vi "InterceptBall.vi"(6 "passer tactic":T1=enum."PenaltyAttacker", 7 "firstCall":bool, 8 "error in (no error)":errorcluster, 9 "Robot":refnum<class "Robot.lvclass">, 10 "Game":refnum<class "Game.lvclass">, 11 "ShootTactic in":refnum<class "ShootTactic.lvclass">) -> (0 "error out":errorcluster, 2 "robot out":refnum<class "Robot.lvclass">, 3 "ShootTactic out":refnum<class "ShootTactic.lvclass">)   [LabVIEW 2023]
uses:
  Utilities_class/Utilities.lvclass
  WaitBallTrajSkill_class/WaitBallTrajSkill.lvclass
  Robot_class/robotKickToStates.ctl
  Robot_class/tactics.ctl
  Robot_class/roles.ctl
  Robot_class/Robot.lvclass
  Ally_class/Ally.lvclass
  Parameters_class/Parameters.lvclass
  Game_class/Game.lvclass
  Zone_class/Zone.lvclass
  Ball_class/Ball.lvclass
  Field_class/Field.lvclass
  C:/Users/ebert/Desktop/roboime/SSL_AI/Skill_class/Skill.lvclass
  C:/Users/ebert/Desktop/roboime/SSL_AI/WaitBallTrajSkill_class/WaitBallTrajSkill.lvclass
  ShootTactic.lvclass
  C:/Users/ebert/Desktop/roboime/SSL_AI/Tactic_class/Tactic.lvclass
  C:/Users/ebert/Desktop/roboime/SSL_AI/ShootTactic_class/ShootTactic.lvclass
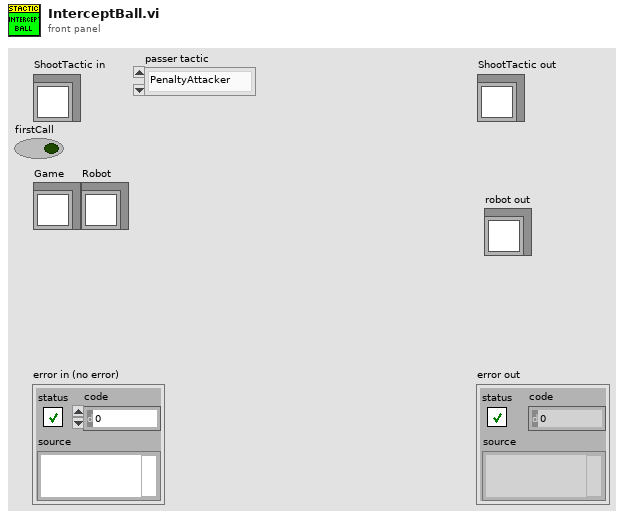
[diagram p1: front panel]
types:
  T1 = typedef "tactics.ctl" = enum16{"GoToBallPlacementPosition", "PlaceBall", "GoToBallPlacement", "5Robots", "BallPlacementEnemy", "ReceivePassInFuturePoint", "Roller", "PrepareRollToPassRollerGoTo", "PrepareRollToPassReceiverGoTo", "WaitRoll", "PositionToRoll", "PenaltyAttacker", "PassObserver", "PenaltyDefense", "TableReceiverTactic", "Test", "DefendGoal", "Marker", "FollowAttacker", "DefendArea", "Shoot", "AttackerAimGoal", "AttackerBallOutOfField", "AttackerBlock", "AttackerStop", "Duelist", "Halt", "ZigZag", "GoTo", "Timeout", "KickToBestRobot", "KickToPassReceiver", "PositionToReceivePass", "WaitPass", "GoToTarget"}
  T2 = typedef "roles.ctl" = enum16{"SimpleBallPlacement", "BallPlacementAllyPasser", "BallPlacementAllyReceiver", "BallPlacementEnemy", "5Robots5th", "PassBestReceiver", "5Robots4th", "5Robots3rd", "5Robots2nd", "5Robots1st", "PassBestRobot", "WaitPass", "ABCThirdKicker", "ABCFirstKicker", "ABCSecondKicker", "Tabler", "TableFinalizer", "PrepareRollToPassRoller", "PrepareRollToPassReceiver", "SimplePassRoll", "SimplePassRollReceiver", "PenaltyDefense", "PreparePassReceiver 2", "PreparePassReceiver 1", "PassObserver", "Timeout", "Goto", "ZigZag", "None", "BallOutOfField", "DefenderArea", "Duelist", "AttackerStop", "FollowAttacker", "KeeperRole", "KickPenalty", "AttackerAimGoal", "AttackerBlock", "Marker", "Halt", "Shoot", "PassKicker", "PassReceiver", "TestRole", "PenaltyAttacker"}
  T3 = typedef "robotKickToStates.ctl" = enum16{"shootFromDirect", "avoidCollideBall", "goToBackBall", "none", "walk", "turn", "turnAntiClockWise", "turnClockwise", "oldKickToShoot", "oldKickToGoToBackBall", "shoot"}
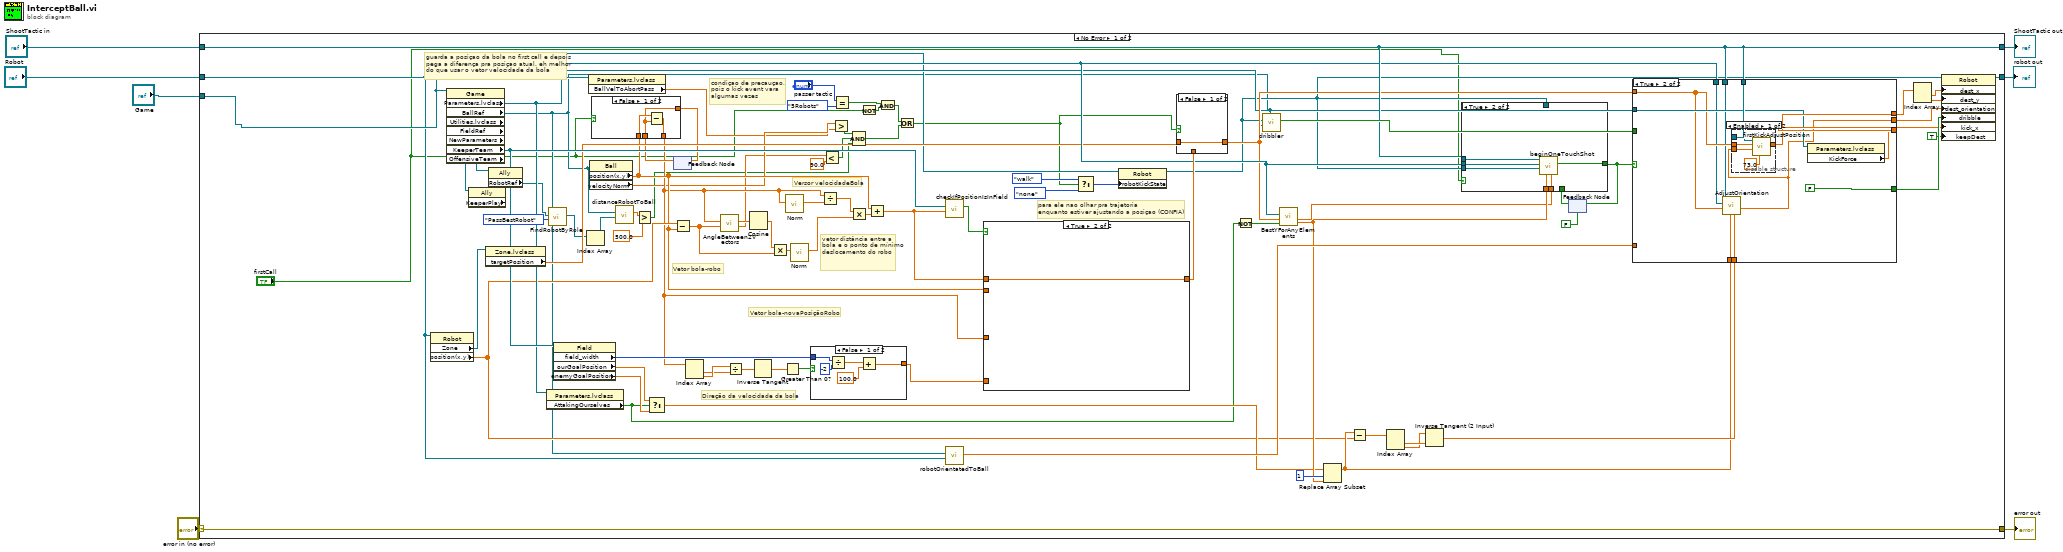
[diagram p0: block diagram]
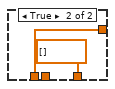
[diagram p2: hidden frame]
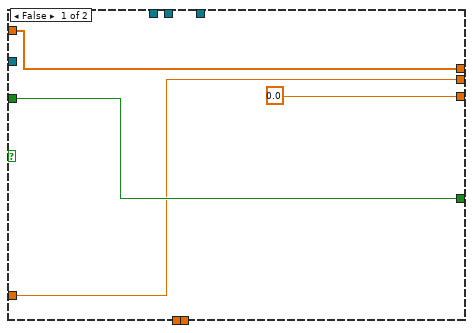
[diagram p4: hidden frame]
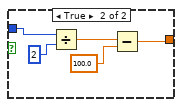
[diagram p7: hidden frame]
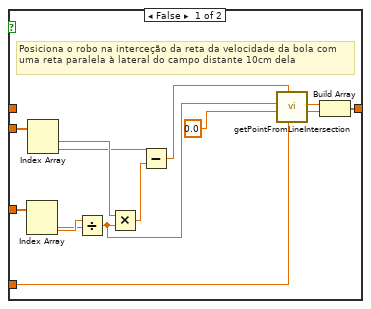
[diagram p8: hidden frame]
diagram:
  n1 = case shown="No Error" "error in (no error)" {
    selector: "error in (no error)" -> [w93 w155]
    tunnel: [w93 w155] -> w6
    tunnel: [w56 w154] -> w4
    tunnel: "ShootTactic in" -> [w56 w154]
    tunnel: "Robot" -> [w40 _]
    tunnel: "Game" -> [w55 _]
    tunnel: [w92 _] -> w2
    frame No Error {
      # "guarda a posiçao da bola no first call e depois\npega a diferença pra posiçao atual. eh melhor\ndo que usar o vetor velocidade da bola"
      # "condiçao de precauçao,\npois o kick event vara \nalgumas vezes"
      # "para ele nao olhar pra trajetoria \nenquanto estiver ajustando a posiçao (CONFIA)"
      # "vetor distância entre a bola e o ponto de mínimo deslocamento do robo"
      # "Versor velocidadeBola"
      # "Direção da velocidade da bola"
      # "Vetor bola-novaPosiçãoRobo"
      # "Vetor bola-robo"
      n2 = property class="Robot"(reference=w40) -> ("Zone"=w43:refnum<class "Zone.lvclass">, "position(x,y)"=w44:dbl[])  [unwired: 1 in, 2 out]
      n3 = property class="Game" props=["Parameters.lvclass", "BallRef", "Utilities.lvclass", "FieldRef", "NewParameters", "KeeperTeam", "OffensiveTeam"](reference=w55) -> ("Parameters.lvclass"=w45:refnum<class "Parameters.lvclass">, "BallRef"=w12:refnum<class "Ball.lvclass">, "FieldRef"=w78:refnum<class "Field.lvclass">, "KeeperTeam"=w68:refnum<class "Ally.lvclass">, "OffensiveTeam"=w16:refnum<class "Ally.lvclass">)  [unwired: 1 in, 4 out]
      n4 = property class="Ally" props=["KeeperPlay"](reference=w68) -> ()  [unwired: 1 in, 3 out]
      n5 = property class="Zone.lvclass"(reference=w43) -> ("targetPosition"=w42:dbl[])  [unwired: 1 in, 2 out]
      n6 = property class="Ally"(reference=w16) -> ("RobotRef"=w15:refnum<class "Robot.lvclass">[])  [unwired: 1 in, 2 out]
      n7 = property class="Parameters.lvclass"(reference=w45) -> ("AttakingOurselves"=w49:bool)  [unwired: 1 in, 2 out]
      n8 = call "FindRobotByRole.vi"("role"=roles."PassBestRobot", "RobotRef"=w15) -> ("Robots"=w14:refnum<class "Robot.lvclass">[])  [unwired: 6 in, 3 out]
      n9 = property class="Field"(reference=w78) -> ("field_width"=w69:i32, "ourGoalPosition"=w52:dbl[], "enemyGoalPosition"=w51:dbl[])  [unwired: 1 in, 2 out]
      n10 = Index Array(array=w14) -> (element=w13:refnum<class "Robot.lvclass">)  [unwired: 1 in]
      n11 = property class="Parameters.lvclass"(reference=w45) -> ("BallVelToAbortPass"=w23:dbl)  [unwired: 1 in, 2 out]
      n12 = property class="Ball"(reference=w12) -> ("position(x,y)"=w31:dbl[], "velocityNorm"=w24:dbl)  [unwired: 1 in, 2 out]
      n13 = call "distanceRobotToBall.vi"("Robot"=w13, "Ball"=w12) -> ("Distance Robot To Ball"=w11:dbl)  [unwired: 7 in, 2 out]
      n14 = Greater?(x=w11, y=500.0) -> (0:w9:bool)
      n15 = Select(t=w52, s=w49, f=w51) -> (s? t:f=w50:dbl[])
      n16 = feedback #1() -> (w30:dbl[])  [unwired: 1 in]
      n17 = case shown="False" "firstCall" {
        tunnel: w31 -> [w96 w98]
        tunnel: w30 -> [w95 _]
        tunnel: [w95 w98] -> w29
        tunnel: [w94 dbl[] []] -> w27
        frame False {
          n18 = Subtract(x=w96, y=w95) -> (x-y=w94:dbl[])
        }
        frame True {
        }
      }
      n19 = feedback-in #1(w29) -> ()
      n20 = Subtract(x=w44, y=w31) -> (x-y=w41:dbl[])
      n21 = Index Array(array=w27) -> (element #1=w87:dbl, element #2=w88:dbl)  [unwired: 2 in]
      n22 = call "AngleBetween2Vectors.vi"("Array 1"=w41, "Array 2"=w27) -> ("angleInDegrees"=w18:dbl, "angleInRadians(default)"=w46:dbl)  [unwired: 6 in, 2 out]
      n23 = Divide(x=w88, y=w87) -> (x/y=w86:dbl)
      n24 = Cosine(x=w46) -> (cos(x)=w91:dbl)
      n25 = Inverse Tangent(1:w86) -> (0:w61:dbl)
      n26 = Multiply(x=w91, y=w41) -> (x*y=w82:dbl[])
      n27 = Greater Than 0?(x=w61) -> (x > 0?=w85:bool)
      n28 = call "Norm.vi"("2D vector"=w27) -> ("Modulo"=w28:dbl)  [unwired: 8 in, 2 out]
      n29 = call "Norm.vi"("2D vector"=w82) -> ("Modulo"=w79:dbl)  [unwired: 8 in, 2 out]
      n30 = case shown="False" w85 {
        tunnel: [w132 w137] -> w84
        tunnel: w69 -> [w129 w134]
        frame False {
          n31 = Divide(x=w129, y=-2) -> (x/y=w131:dbl)
          n32 = Add(x=w131, y=100.0) -> (x+y=w132:dbl)
        }
        frame True {
          n33 = Divide(x=w134, y=2) -> (x/y=w136:dbl)
          n34 = Subtract(x=w136, y=100.0) -> (x-y=w137:dbl)
        }
      }
      n35 = Divide(x=w27, y=w28) -> (x/y=w80:dbl[])
      n36 = Less?(x=w18, y=90.0) -> (x < y?=w20:bool)
      n37 = Greater?(x=w24, y=w23) -> (0:w22:bool)
      n38 = Equal?(x="passer tactic", y=tactics."5Robots") -> (x = y?=w33:bool)
      n39 = Multiply(x=w80, y=w79) -> (x*y=w81:dbl[])
      n40 = Compound Arithmetic op=AND(w22, w20, w9) -> (w21:bool)
      n41 = Not(x="firstCall") -> (.not. x?=w32:bool)
      n42 = Add(x=w31, y=w81) -> (x+y=w89:dbl[])
      n43 = And(x=w33, y=w32) -> (x .and. y?=w26:bool)
      n44 = Or(x=w26, y=w21) -> (x .or. y?=w25:bool)
      n45 = call "checkIfPositionIsInField.vi"("Position"=w89, "FieldRef"=w78) -> ("Position Is In Field?"=w90:bool)  [unwired: 5 in, 4 out]
      n46 = call "robotOrientatedToBall.vi"("Robot"=w40, "BallRef"=w12) -> ("Orientation"=w73:dbl)  [unwired: 7 in, 2 out]
      n47 = case shown="True" w90 {
        tunnel: w89 -> [_ w153]
        tunnel: [w150 w153] -> w83
        tunnel: w84 -> [w148 _]
        tunnel: w31 -> [w147 _]
        tunnel: w27 -> [w146 _]
        frame False {
          # "Posiciona o robo na interceção da reta da velocidade da bola com uma reta paralela à lateral do campo distante 10cm dela"
          n48 = Index Array(array=w146) -> (element #1=w144:dbl, element #2=w145:dbl)  [unwired: 2 in]
          n49 = Index Array(array=w147) -> (element #1=w143:dbl, element #2=w142:dbl)  [unwired: 2 in]
          n50 = Divide(x=w145, y=w144) -> (x/y=w139:dbl)
          n51 = Multiply(x=w143, y=w139) -> (x*y=w141:dbl)
          n52 = Subtract(x=w142, y=w141) -> (x-y=w140:dbl)
          n53 = call "getPointFromLineIntersection.vi"("b2"=w148, "b1"=w140, "a2"=0.0, "a1"=w139) -> ("y_intersection"=w151:dbl, "x_intersection"=w152:dbl)  [unwired: 4 in, 2 out]
          n54 = Build Array(w152, w151) -> (w150:dbl[])
        }
        frame True {
        }
      }
      n55 = Select(t=robotKickToStates."walk" ("robotKickState"), s=w25, f=robotKickToStates."none" ("robotKickState")) -> (s? t:f=w36:T3)
      n56 = property class="Robot"(reference=w40, "robotKickState"=w36) -> (reference out=w39:refnum<class "Robot.lvclass">)  [unwired: 1 in, 1 out]
      n57 = case shown="False" w25 {
        tunnel: w83 -> [_ w128]
        tunnel: [w127 w128] -> w54
        tunnel: w42 -> [w127 _]
        frame False {
        }
        frame True {
        }
      }
      n58 = Not(x=w49) -> (.not. x?=w48:bool)
      n59 = call "dribbler.vi"("Parameters.lvclass"=w45, "Ball"=w12, "Robot"=w39) -> ("Dribbler?"=w76:bool)  [unwired: 6 in, 2 out]
      n60 = call "BestYForAnyElements.vi"("inimigos"=w48, "Position to be analyzed"=w54, "Game"=w55) -> ("Best y"=w53:dbl, "Gap Coord"=w47:dbl[])  [unwired: 5 in, 2 out]
      n61 = Replace Array Subset(array=w50, new element=w53, index=1) -> (w57:dbl[])
      n62 = Subtract(x=w57, y=w44) -> (x-y=w70:dbl[])
      n63 = Index Array(array=w70) -> (element #1=w72:dbl, element #2=w71:dbl)  [unwired: 2 in]
      n64 = Inverse Tangent (2 Input)(1:w72, 2:w71) -> (0:w58:dbl)
      n65 = feedback #2(FALSE ("Boolean")) -> (w63:bool)
      n66 = case shown="True" "firstCall" {
        tunnel: w56 -> [_ w105]
        tunnel: w55 -> [_ w104]
        tunnel: w39 -> [_ w103]
        tunnel: [w99 w102] -> w64
        tunnel: w63 -> [w99 _]
        tunnel: w39 -> [_ _]
        tunnel: w53 -> [_ w101]
        tunnel: w47 -> [_ w100]
        frame False {
        }
        frame True {
          n67 = call "beginOneTouchShot.vi"("Gap Coord"=w100, "bestY"=w101, "Robot"=w103, "Game"=w104, "WaitBallTrajSkill in"=w105) -> ("Boolean"=w102:bool)  [unwired: 4 in, 2 out]
        }
      }
      n68 = feedback-in #2(w64) -> ()
      n69 = case shown="True" w64 {
        tunnel: [w109 FALSE ("Dribbler?")] -> w77
        tunnel: w76 -> [w109 _]
        tunnel: [w108 w110] -> w75
        tunnel: w73 -> [w108 _]
        tunnel: [0.0 ("kick_x") w116] -> w74
        tunnel: w45 -> [_ w117]
        tunnel: w56 -> [_ w119]
        tunnel: w54 -> [w106 w113]
        tunnel: [w106 w118] -> w67
        tunnel: w58 -> [_ w115]
        tunnel: w57 -> [_ w114]
        tunnel: w55 -> [_ w112]
        tunnel: w56 -> [_ w111]
        frame False {
        }
        frame True {
          n70 = call "AdjustOrientation.vi"("orientation"=w115, "target"=w114, "dest"=w113, "Game"=w112, "WaitBallTrajSkill in"=w111) -> ("orientation out"=w110:dbl)  [unwired: 4 in, 2 out]
          n71 = disable-structure shown="Enabled" {
            disable-tunnel: w119 -> [w125 _]
            disable-tunnel: [w124 w126] -> w118
            disable-tunnel: w113 -> [w122 w126]
            disable-tunnel: w110 -> [w121 _]
            frame Enabled {
              n72 = call "firstKickAdjustPosition.vi"("Dist"=73.0, "Orientation"=w121, "Dest"=w122, "WaitBallTrajSkill in"=w125) -> ("AdjustDest"=w124:dbl[])  [unwired: 5 in, 2 out]
            }
            frame Disabled {
            }
          }
          n73 = property class="Parameters.lvclass"(reference=w117) -> ("KickForce"=w116:dbl)  [unwired: 1 in, 2 out]
        }
      }
      n74 = Index Array(array=w67) -> (element #1=w65:dbl, element #2=w66:dbl)  [unwired: 2 in]
      n75 = property class="Robot"(reference=w39, "dest_x"=w65, "dest_y"=w66, "dest_orientation"=w75, "dribble"=w77, "kick_x"=w74, "keepDest"=TRUE) -> (reference out=w92:refnum<class "Robot.lvclass">)  [unwired: 1 in, 1 out]
    }
    frame Error {
    }
  }
  "error out" <- w6
  "ShootTactic out" <- w4
  "robot out" <- w2
